vi "Receive Messages from Azure Queue.vi"() -> ()   [LabVIEW 2015]
doc: "Demonstrates how to receive messages from an existing Azure queue."
uses:
  Core/Azure Credentials.ctl
  Core/NI_Azure_Core.lvlib
  Core/Session/Session.lvclass
  Queue/NI_Azure_Queue.lvlib
panel:
  out "Messages":i32(listbox)
  in  "Access Key":string
  in  "Storage Account Name":string
  in  "Queue Name":string
  # "Overview: Demonstrates how to receive messages from an existing Azure queue.\nRequirements: NI Cloud Toolkit for Azure and a registered Microsoft Azure account\nInstructions:\n1. Specify the Storage Account Name and Access Key for your Azure account. You can create an account at http://azure.microsoft.com.\n2. Specify a Queue Name for the queue from which you want to receive messages.\n3. Run the VI. Messages associated with your queue should be listed in the Messages indicator. Note that a single call of the Get Messages VI can return a maximum of 32 messages from the queue."
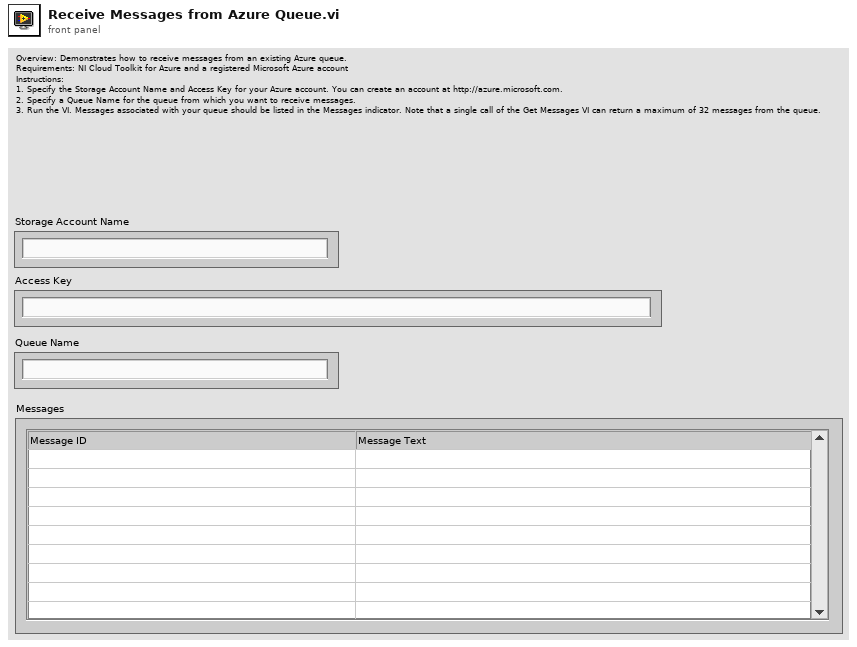
[diagram p1: front panel]
types:
  T1 = typedef "NI_Azure_Core.lvlib/Azure Credentials.ctl" = cluster{"Storage Account Name":string, "Access Key":string}
  T2 = typedef "NI_Azure_Queue.lvlib/Message.ctl" = cluster{"Message ID":string, "Insertion Time":string, "Expiration Time":string, "Pop Receipt":string, "Time Next Visible":string, "Dequeue Count":i32, "Message Text":string}
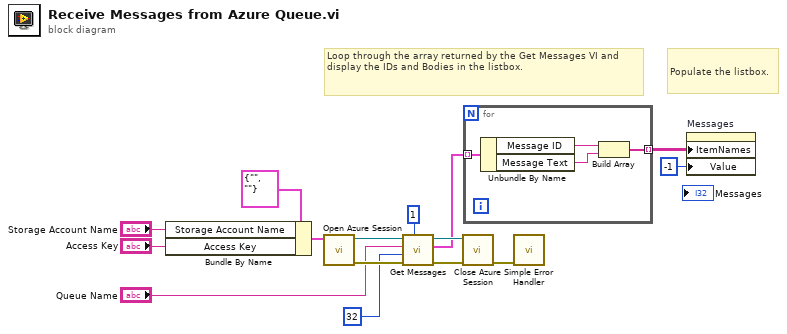
[diagram p0: block diagram]
diagram:
  # "Loop through the array returned by the Get Messages VI and display the IDs and Bodies in the listbox."
  # "Populate the listbox."
  n1 = Bundle By Name(cluster=T1 {"Storage Account Name"="", "Access Key"=""} ("Credentials"), "Storage Account Name"="Storage Account Name", "Access Key"="Access Key") -> (w12:T1)
  n2 = call "Open Azure Session.vi"("Credentials"=w12) -> ("error out"=w10:errorcluster, "Azure Session"=w11:refnum<class "Session.lvclass">)  [unwired: 9 in]
  n3 = call "Get Messages.vi"("Visibility timeout (30 seconds)"=u32 1, "error in (no error)"=w10, "Number of messages (1)"=u32 32, "Queue"="Queue Name", "Azure Session in"=w11) -> ("error out"=w6:errorcluster, "Messages"=w4:T2[], "Azure Session out"=w5:refnum<class "Session.lvclass">)  [unwired: 4 in]
  n4 = call "Close Azure Session.vi"("error in (no error)"=w6, "Azure Session"=w5) -> ("error out"=w3:errorcluster)  [unwired: 9 in]
  n5 = for {
    tunnel: w4 -> [w19] mode=indexing
    tunnel: [w16] -> w2 mode=indexing
    n6 = Unbundle By Name(w19) -> ("Message ID"=w17:string, "Message Text"=w18:string)
    n7 = Build Array(w17, w18) -> (w16:string[])
  }
  n8 = call <vilib>:"Simple Error Handler.vi"("error in (no error)"=w3) -> ()  [unwired: 4 in, 5 out]
  n9 = property on="Messages" class="MCListbox (strict)"("ItemNames"=w2, "Value"=-1 ("Messages")) -> ()  [unwired: 2 in, 2 out]
